vi "Untitled 3.vi"   [LabVIEW 2018]
uses:
  Classes/Controller/Controller.lvclass
  Classes/Controller/Motion/Motion.lvclass
  C:/Users/hep/Documents/CMU gantry/Classes/Controller/Controller.lvclass
types:
  T1 = typedef "Controller.lvclass/Controllers.ctl" = cluster{"I-O.lvclass":refnum<class "I-O.lvclass">, "Gantry":refnum<k24>, "Dispenser":refnum<visa-resource-name>}
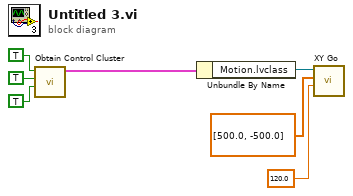
[diagram p0: block diagram]
diagram:
  n1 = call "Obtain Control Cluster.vi"("I/O"=TRUE, "Dispense"=TRUE, "Motion"=TRUE) -> ("Control Out"=w4:T1)  [unwired: 8 in]
  n2 = Unbundle By Name(w4) -> ("Motion.lvclass"=w3:refnum<class "Motion.lvclass">)
  n3 = call "XY Go.vi"("Speed"=120.0, "XY In"=dbl[] [500.0, -500.0] ("XY"), "Gantry In"=w3) -> ()  [unwired: 6 in, 3 out]
